vi "IMAQ Stack to xyzct and KLB Data Type.vi"(8 "error in":errorcluster, 11 "IMAQ Stack":T1[](array[typedef])) -> (0 "error out":errorcluster, 2 "KLB Data Type":u8, 3 "XYZCT":u32[](array[numeric]))   [LabVIEW 2013, in "KLB.lvlib"]
doc: "Looks at first element in array, array size, and pixel depth and outputs xyzct array and data type for KLB compression functions.\n\nInputs\nIMAQ Stack (Required)\n\nOutputs\nxyzct array for KLB Library function\nData Type for KLB Library function"
uses:
  KLB.lvlib
  <vilib>/vision/Image Controls.llb/IMAQ Image.ctl
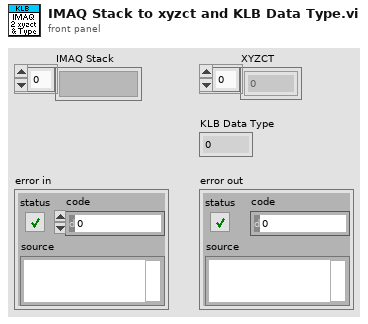
[diagram p1: front panel]
types:
  T1 = typedef "IMAQ Image.ctl" = refnum<image>
  T2 = typedef "Image Type" = u32
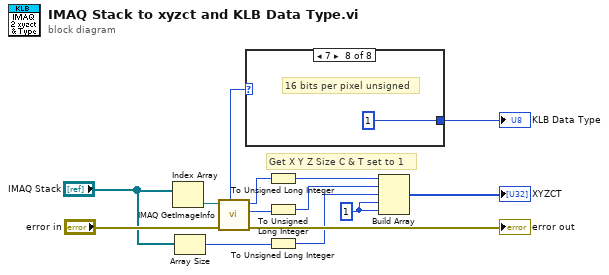
[diagram p0: block diagram]
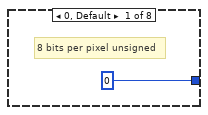
[diagram p2: hidden frame]
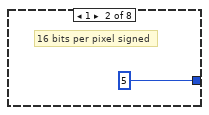
[diagram p3: hidden frame]
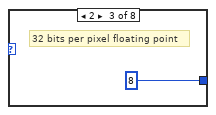
[diagram p4: hidden frame]
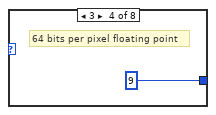
[diagram p5: hidden frame]
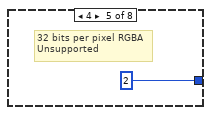
[diagram p6: hidden frame]
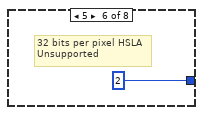
[diagram p7: hidden frame]
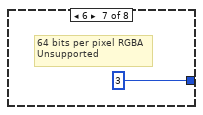
[diagram p8: hidden frame]
diagram:
  w7 = u32 1 ("element")
  # "Get X Y Z Size C & T set to 1"
  n1 = Index Array(array="IMAQ Stack") -> (element=w8:T1)  [unwired: 1 in]
  n2 = Array Size(array="IMAQ Stack") -> (size(s)=w3:i32)
  n3 = call "IMAQ GetImageInfo"("error in (no error)"="error in", "Image"=w8) -> ("error out"=→"error out":errorcluster, "Y Resolution"=w11:i32, "X Resolution"=w10:i32, "Image Type"=w12:T2)  [unwired: 2 in, 4 out]
  n4 = case shown="7" w12 {
    tunnel: [u8 0 u8 5 u8 8 u8 9 u8 2 u8 2 u8 3 u8 1] -> w1
    frame 0, Default {
      # "8 bits per pixel unsigned"
    }
    frame 1 {
      # "16 bits per pixel signed"
    }
    frame 2 {
      # "32 bits per pixel floating point"
    }
    frame 3 {
      # "64 bits per pixel floating point"
    }
    frame 4 {
      # "32 bits per pixel RGBA\nUnsupported"
    }
    frame 5 {
      # "32 bits per pixel HSLA\nUnsupported"
    }
    frame 6 {
      # "64 bits per pixel RGBA\nUnsupported"
    }
    frame 7 {
      # "16 bits per pixel unsigned"
    }
  }
  "KLB Data Type" <- w1
  n5 = To Unsigned Long Integer(number=w10) -> (unsigned 32bit integer=w4:u32)
  n6 = To Unsigned Long Integer(number=w11) -> (unsigned 32bit integer=w5:u32)
  n7 = To Unsigned Long Integer(number=w3) -> (unsigned 32bit integer=w6:u32)
  n8 = Build Array(w4, w5, w6, w7, w7) -> (→"XYZCT":u32[])
